vi "Creator Queue Alias.vi"(11 "Hello World Queue in":refnum<class "Hello World Queue.lvclass">) -> (2 "Creator Queue Alias":string, 3 "Hello World Queue out":refnum<class "Hello World Queue.lvclass">)   [LabVIEW 2021, in "Hello World Queue.lvlib" / "Hello World Queue.lvclass"]
uses:
  Hello World Queue.lvclass
  Hello World Queue.lvclass/Hello World Queue.ctl
  jettl/Queue jettl/Queue jettl.lvclass
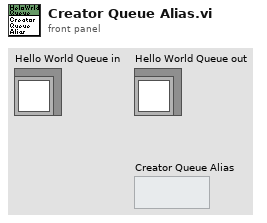
[diagram p1: front panel]
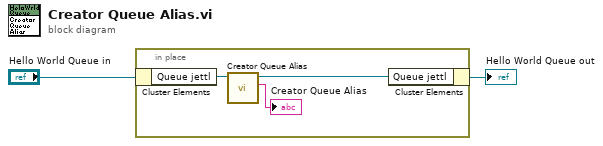
[diagram p0: block diagram]
diagram:
  n1 = in-place {
    n2 = in-place-cluster #1("Hello World Queue in") -> ("Queue jettl"=w5:refnum<class "Queue jettl.lvclass">)
    n3 = call-dynamic "Creator Queue Alias.vi"("Queue jettl in"=w5) -> ("Creator Queue Alias"=→"Creator Queue Alias":string, "Queue jettl out"=w4:refnum<class "Queue jettl.lvclass">)  [unwired: 9 in]
    n4 = in-place-cluster #1("Queue jettl"=w4) -> (→"Hello World Queue out":refnum<class "Hello World Queue.lvclass">)
  }
